vi "Get Device User ID.vi"(8 "Error In":errorcluster, 11 "LINX Resource":T1) -> (0 "Error Out":errorcluster, 2 "Device User ID":u16, 3 "LINX Resource":T1)   [LabVIEW 2014, in "LMH-LINX.lvlib"]
doc: "Get the numeric user ID of the LINX device. This is a user configurable value and defaults to 0 when it has not been set."
uses:
  <vilib>/MakerHub/LINX/LMH-LINX.lvlib
  <vilib>/MakerHub/LINX/Private/Type Defs/LINX Ref.ctl
  <vilib>/MakerHub/LINX/Private/Type Defs/Platform.ctl
  <vilib>/MakerHub/LINX/Private/Type Defs/Interface.ctl
  <vilib>/MakerHub/LINX/Private/Device/Type Defs/LINX Device Config.ctl
  <vilib>/MakerHub/LINX/Private/Device/Type Defs/TCP Config.ctl
  <vilib>/MakerHub/LINX/Private/Device/Type Defs/Channels.ctl
  <vilib>/MakerHub/LINX/Private/Type Defs/Error Type.ctl
  <vilib>/MakerHub/LINX/Private/Device/Device.lvlib
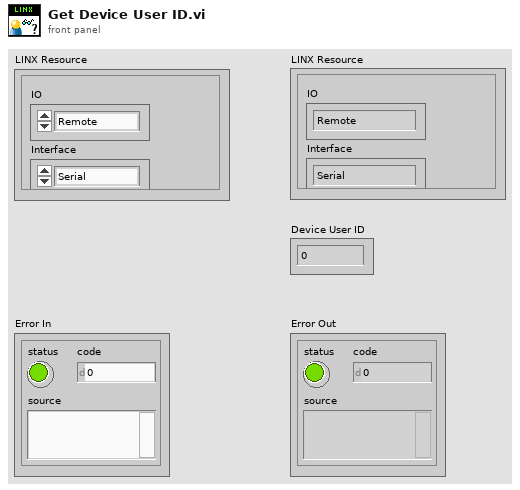
[diagram p1: front panel]
types:
  T1 = typedef "LMH-LINX.lvlib/LINX Ref.ctl" = cluster{"IO":T2, "Interface":T3, "LINX Device Config":T4}
  T2 = typedef "LMH-LINX.lvlib/Platform.ctl" = enum16{"Remote", "Local"}
  T3 = typedef "LMH-LINX.lvlib/Interface.ctl" = enum16{"Serial", "TCP"}
  T4 = typedef "LMH-LINX.lvlib/Device.lvlib/LINX Device Config.ctl" = cluster{"Interface":T3, "COM Port":refnum<visa-resource-name>, "TCP Configuration":T5, "Device Family":u8, "Device ID":u8, "Device Name":string, "TCP Ref":refnum<k5>, "Channels":T6}
  T5 = typedef "LMH-LINX.lvlib/Device.lvlib/TCP Config.ctl" = cluster{"IP Address":string, "Port":u16}
  T6 = typedef "LMH-LINX.lvlib/Channels.ctl" = cluster{"DI":u8[], "DO":u8[], "AI":u8[], "AO":u8[], "PWM":u8[], "QE":u8[], "UART":u8[], "I2C 2":u8[], "SPI":u8[], "CAN":u8[], "Servo":u8[], "AI Ref (V)":dbl, "AI Resolution (Bits)":u8, "AO Ref (V)":dbl, "AO Resolution (Bits)":u8}
  T7 = typedef "LMH-LINX.lvlib/Error Type.ctl" = enum16{"Unknown", "Timeout", "Corrupt Return Packet", "Unable To Connect", "Command Not Supported", "Channel DNE", "Invalid COM Config", "Firmware Version Mismatch", "myRIO Support", "CMD Specific Error", "Local IO Not Supported"}
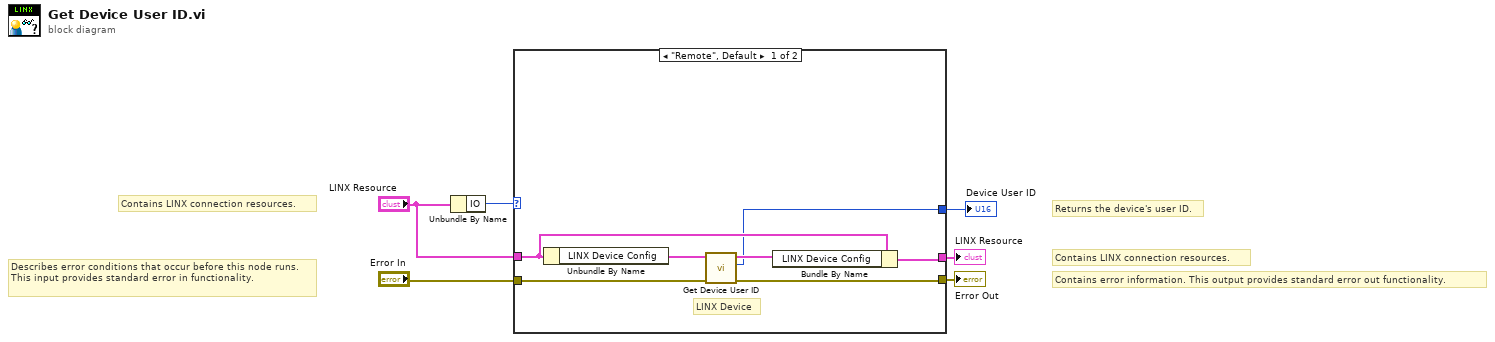
[diagram p0: block diagram]
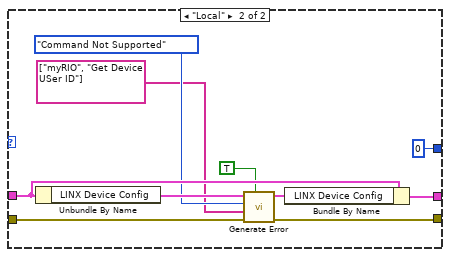
[diagram p2: hidden frame]
diagram:
  # "Returns the device's user ID."
  # "Contains LINX connection resources."
  # "Contains error information. This output provides standard error out functionality."
  # "Contains LINX connection resources."
  # "Describes error conditions that occur before this node runs. This input provides standard error in functionality."
  n1 = Unbundle By Name("LINX Resource") -> ("IO"=w6:T2)
  n2 = case shown="\"Remote\", Default" w6 {
    tunnel: [w8 w19] -> w5
    tunnel: [w13 w18] -> w2
    tunnel: "Error In" -> [w9 w20]
    tunnel: "LINX Resource" -> [w12 w23]
    tunnel: [w7 u16 0 ("Device User ID")] -> w1
    frame "Remote", Default {
      # "LINX Device"
      n3 = Unbundle By Name(w12) -> ("LINX Device Config"=w10:T4)
      n4 = call <vilib>:"Get Device User ID.vi"("Error In"=w9, "LINX Device Config"=w10) -> ("Error Out"=w8:errorcluster, "Device User ID"=w7:u16, "LINX Device Config"=w11:T4)  [unwired: 7 in]
      n5 = Bundle By Name(cluster=w12, "LINX Device Config"=w11) -> (w13:T1)
    }
    frame "Local" {
      n6 = Unbundle By Name(w23) -> ("LINX Device Config"=w22:T4)
      n7 = call <vilib>:"Generate Error.vi"("Is Warning? (False)"=TRUE, "Error In"=w20, "Arguments"=string[] ["myRIO", "Get Device USer ID"], "Error Type"=Error_Type."Command Not Supported", "LINX Device Config"=w22) -> ("Error Out"=w19:errorcluster, "Dup LINX Device Config"=w21:T4)  [unwired: 5 in]
      n8 = Bundle By Name(cluster=w23, "LINX Device Config"=w21) -> (w18:T1)
    }
  }
  "Error Out" <- w5
  "LINX Resource" <- w2
  "Device User ID" <- w1
